vi "BtnFacade.vi"(0 "Data In":T5={"Btn"=FALSE, "Microprocessor"={"VISA Refnum in"="", "All Code"="Hi"}}, 2 "Display State In":T3, 3 "Container State":T4) -> (6 "Data Out":T5={"Btn"=FALSE, "Microprocessor"={"VISA Refnum in"="", "All Code"="Hi"}}, 7 "Display State Out":T3, 8 "Action":T2)   [LabVIEW 2016, in "BtnXControl.xctl"]
uses:
  BtnXControl.xctl
  <vilib>/_xctls/Action.ctl
  <vilib>/_xctls/XControlSupport.lvlib
  <vilib>/_xctls/Container State.ctl
  BtnData.ctl
  BtnState.ctl
  uPythonX/PythonData.ctl
  uPythonX/uPythonX.xctl
panel:
  in  "Microprocessor":T1={"VISA Refnum in"="", "All Code"="Hi"}
  in  "Settings":bool
  in  "Boolean":bool
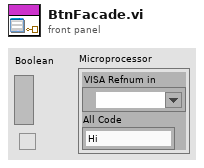
[diagram p1: front panel]
types:
  T1 = typedef "uPythonX.xctl/PythonData.ctl" = cluster{"VISA Refnum in":refnum<visa-resource-name>, "All Code":string}
  T2 = typedef "XControlSupport.lvlib/Action.ctl" = cluster{"Data Changed?":bool, "State Changed?":bool, "Action Name":string}
  T3 = typedef "BtnXControl.xctl/BtnState.ctl" = cluster{"Numeric":dbl}
  T4 = typedef "XControlSupport.lvlib/Container State.ctl" = cluster{"Indicator?":bool, "Run Mode?":bool, " Refnum":refnum<vi>}
  T5 = typedef "BtnXControl.xctl/BtnData.ctl" = cluster{"Btn":bool, "Microprocessor":T1}
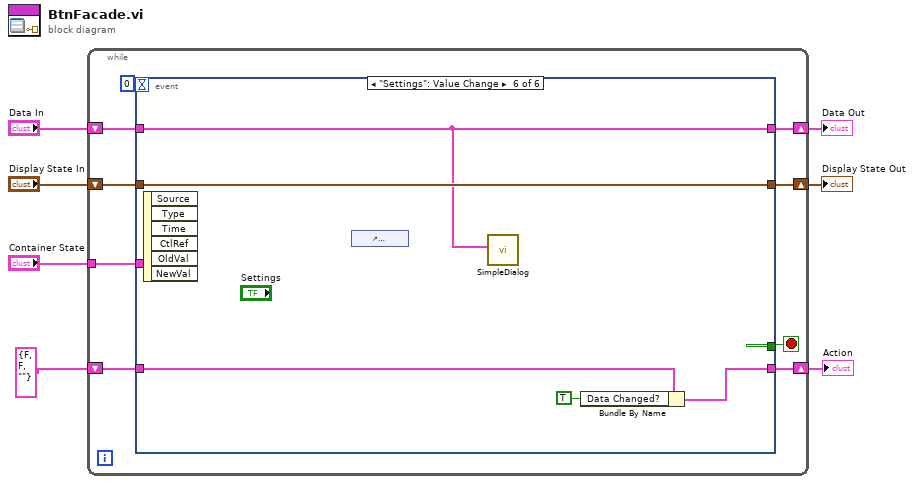
[diagram p0: block diagram]
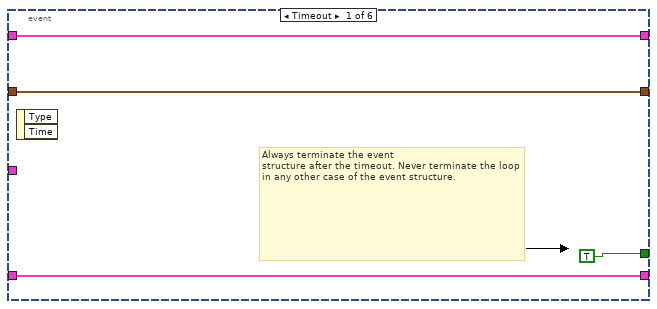
[diagram p2: hidden frame]
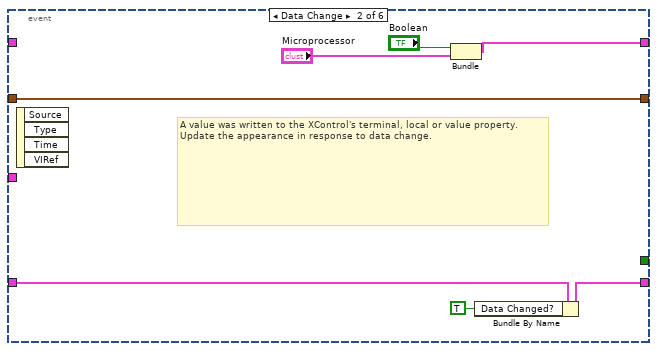
[diagram p3: hidden frame]
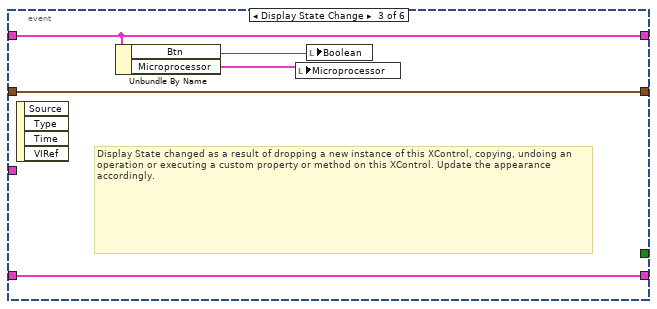
[diagram p4: hidden frame]
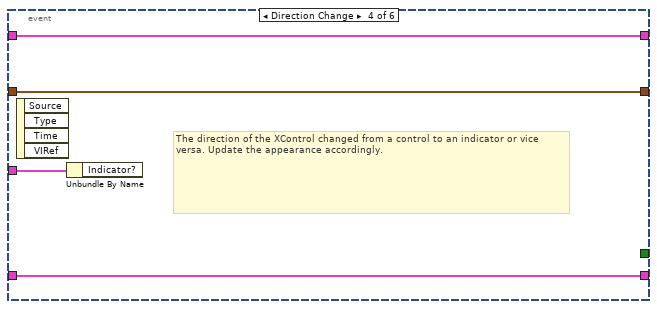
[diagram p5: hidden frame]
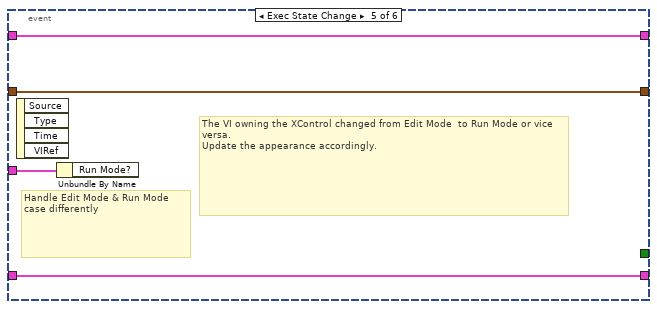
[diagram p6: hidden frame]
diagram:
  n1 = while {
    shift-right: [w15] -> w4
    shift-left: "Display State In" -> [w16]
    tunnel: "Container State" -> [w12]
    shift-right: [w10] -> w7
    shift-left: "Data In" -> [w11]
    shift-right: [w8] -> w2
    shift-left: T2 {"Data Changed?"=FALSE, "State Changed?"=FALSE, "Action Name"=""} ("Action") -> [w9]
    stop <- w14 stop-if-true
    n2 = event shown="[5] \"Settings\": Value Change" {
      selector: _ -> [_ _ _ _ _ _]
      dyn-events: _ -> [_ _ _ _ _ _]
      timeout: 0 -> [_ _ _ _ _ _]
      tunnel: w16 -> [w18 w27 w32 w35 w39 w45]
      tunnel: [w18 w27 w32 w35 w39 w45] -> w15
      tunnel: [TRUE _ _ _ _ _] -> w14
      tunnel: w12 -> [_ _ _ w36 w40 _]
      tunnel: w11 -> [w17 _ w30 w34 w38 w44]
      tunnel: [w17 w21 w30 w34 w38 w44] -> w10
      tunnel: [w19 w25 w31 w33 w37 w41] -> w8
      tunnel: w9 -> [w19 w26 w31 w33 w37 w42]
      event Timeout {
        # "Always terminate the event\nstructure after the timeout. Never terminate the loop in any other case of the event structure."
        n3 = event-data() -> ()  [unwired: 1 in, 2 out]
      }
      event Data Change {
        # "A value was written to the XControl's terminal, local or value property.\nUpdate the appearance in response to data change."
        n4 = event-data() -> ()  [unwired: 1 in, 4 out]
        n5 = Bundle("Boolean"="Boolean", "Microprocessor"="Microprocessor") -> (w21:cluster{"Boolean":bool, "Microprocessor":T1})  [unwired: 1 in]
        n6 = Bundle By Name(cluster=w26, "Data Changed?"=TRUE) -> (w25:T2)
      }
      event Display State Change {
        # "Display State changed as a result of dropping a new instance of this XControl, copying, undoing an operation or executing a custom property or method on this XControl. Update the appearance accordingly."
        n7 = event-data() -> ()  [unwired: 1 in, 4 out]
        n8 = Unbundle By Name(w30) -> ("Btn"=w28:bool, "Microprocessor"=w29:T1)
        n9 = local write "Microprocessor"(w29) -> ()
        n10 = local write "Boolean"(w28) -> ()
      }
      event Direction Change {
        # "The direction of the XControl changed from a control to an indicator or vice versa. Update the appearance accordingly."
        n11 = event-data() -> ()  [unwired: 1 in, 4 out]
        n12 = Unbundle By Name(w36) -> ()  [unwired: 1 out]
      }
      event Exec State Change {
        # "The VI owning the XControl changed from Edit Mode  to Run Mode or vice versa.\nUpdate the appearance accordingly."
        # "Handle Edit Mode & Run Mode\ncase differently"
        n13 = event-data() -> ()  [unwired: 1 in, 4 out]
        n14 = Unbundle By Name(w40) -> ()  [unwired: 1 out]
      }
      event "Settings": Value Change {
        n15 = event-data() -> ()  [unwired: 1 in, 6 out]
        n16 = control-ref of="Microprocessor"() -> ()  [unwired: 1 out]
        n17 = call "SimpleDialog.vi"("Data In"=w44) -> ()  [unwired: 11 in]
        n18 = Bundle By Name(cluster=w42, "Data Changed?"=TRUE) -> (w41:T2)
      }
    }
  }
  "Display State Out" <- w4
  "Data Out" <- w7
  "Action" <- w2
